vi "Check_too_deep.vi"(8 "error in (no error)":errorcluster) -> (0 "error out":errorcluster)   [LabVIEW 2013]
uses:
  My Computer/Controls/EKF_Settings.ctl
  My Computer/Controls/Estimated Position.ctl
  My Computer/Controls/Sensors State.ctl
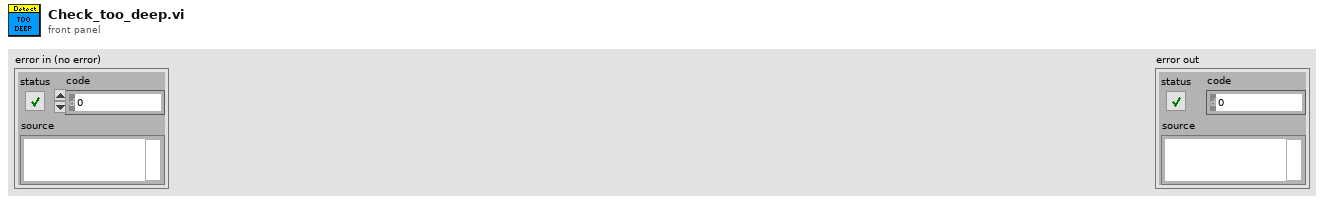
[diagram p1: front panel]
types:
  T1 = typedef "EKF_Settings.ctl" = cluster{"Gravity constant":dbl, "Filter Version":enum16{"IMU Only", "IMU & Pressure", "IMU, Pressure, Compass"}, "Initial Biases":cluster{"Gyro_Bias_nit_x":dbl, "Gyro_Bias_init_y":dbl, "Gyro_Bias_init_z":dbl, "Acc_Bias_init_x":dbl, "Acc_Bias_init_y":dbl, "Acc_Bias_init_z":dbl}, "Use Compass on initialisation":bool, "Initial Biases Covariances":cluster{"Initial_covariance_Gyro_Bias":dbl, "Initial_covariance_Acc_Bias":dbl}, "Magnetic-Field-Vector [utesla]":cluster{"Magf_N_x":dbl, "Magf_N_y":dbl, "Magf_N_z":dbl}, "IMU_Sigmas":cluster{"Sigma_w":dbl, "Sigma_wb":dbl, "Sigma_a":dbl, "Sigma_ab":dbl, "Sigma_m":dbl}, "Measurement Sigmas":cluster{"Sigma_v":dbl, "Sigma_depth":dbl}}
  T2 = enum16{"IMU Only", "IMU & Pressure", "IMU, Pressure, Compass"}
  T3 = typedef "Estimated Position.ctl" = cluster{"X":dbl, "Y":dbl, "Z":dbl, "V_X":dbl, "V_Y":dbl, "V_Z":dbl}
  T4 = typedef "Sensors State.ctl" = cluster{"Leakage-Sensor_enabled":bool, "IMU_enabled":bool, "Swimbladder Fill-State-Sensor_enabled":bool, "Flow-Sensor_enabled":bool, "Depth-Sensor_enabled":bool, "Current-Sensor_enabled":bool, "Calibrate Depth":bool, "SB_Piston_Stuck_Detect_enabled":bool, "Check_too_Deep_enabled":bool}
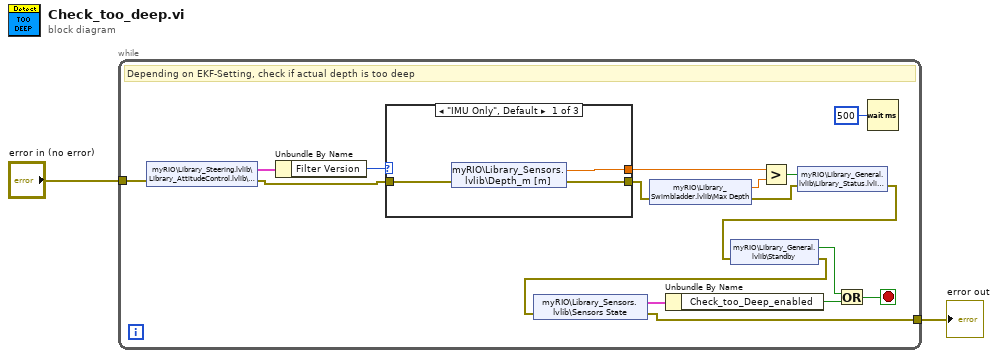
[diagram p0: block diagram]
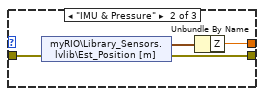
[diagram p2: hidden frame]
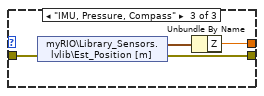
[diagram p3: hidden frame]
diagram:
  n1 = while {
    tunnel: "error in (no error)" -> [w3]
    tunnel: [w4] -> w1
    stop <- w15 stop-if-true
    # "Depending on EKF-Setting, check if actual depth is too deep"
    n2 = shared-variable "myRIO\\Library_Steering.lvlib\\Library_AttitudeControl.lvlib\\EKF_Settings"(error in=w3) -> (w14:T1, error out=w12:errorcluster)
    n3 = Unbundle By Name(w14) -> ("Filter Version"=w13:T2)
    n4 = case shown="\"IMU Only\", Default" w13 {
      tunnel: [w21 w25 w29] -> w11
      tunnel: w12 -> [w22 w24 w27]
      tunnel: [w20 w23 w28] -> w9
      frame "IMU Only", Default {
        n5 = shared-variable "myRIO\\Library_Sensors.lvlib\\Depth_m [m]"(error in=w22) -> (w21:dbl, error out=w20:errorcluster)
      }
      frame "IMU & Pressure" {
        n6 = shared-variable "myRIO\\Library_Sensors.lvlib\\Est_Position [m]"(error in=w24) -> (w26:T3, error out=w23:errorcluster)
        n7 = Unbundle By Name(w26) -> ("Z"=w25:dbl)
      }
      frame "IMU, Pressure, Compass" {
        n8 = shared-variable "myRIO\\Library_Sensors.lvlib\\Est_Position [m]"(error in=w27) -> (w30:T3, error out=w28:errorcluster)
        n9 = Unbundle By Name(w30) -> ("Z"=w29:dbl)
      }
    }
    n10 = shared-variable "myRIO\\Library_Swimbladder.lvlib\\Max Depth"(error in=w9) -> (w10:dbl, error out=w7:errorcluster)
    n11 = Greater?(x=w11, y=w10) -> (0:w8:bool)
    n12 = shared-variable "myRIO\\Library_General.lvlib\\Library_Status.lvlib\\tooDeep"(w8, error in=w7) -> (error out=w5:errorcluster)
    n13 = shared-variable "myRIO\\Library_General.lvlib\\Standby"(error in=w5) -> (w17:bool, error out=w18:errorcluster)
    n14 = shared-variable "myRIO\\Library_Sensors.lvlib\\Sensors State"(error in=w18) -> (w19:T4, error out=w4:errorcluster)
    n15 = Unbundle By Name(w19) -> ("Check_too_Deep_enabled"=w16:bool)
    n16 = Or(x=w17, y=w16) -> (x .or. y?=w15:bool)
    n17 = Wait (ms)(milliseconds to wait=u32 500) -> ()  [unwired: 1 out]
  }
  "error out" <- w1
